vi "Read Is Server.vi"(8 "error in (no error)":errorcluster, 11 "WebSocket Server in":refnum<class "WebSocket Server.lvclass">) -> (0 "error out":errorcluster, 2 "Is Server?":bool, 3 "WebSocket Server out":refnum<class "WebSocket Server.lvclass">)   [LabVIEW 2013, in "WebSockets.lvlib" / "WebSocket Server.lvclass"]
uses:
  WebSocket Server.lvclass
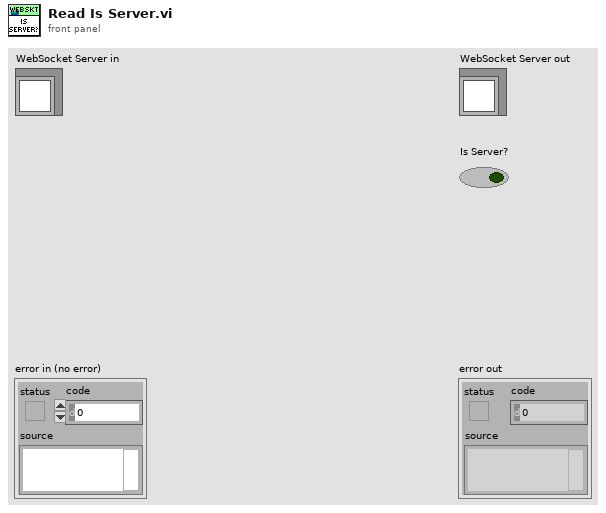
[diagram p1: front panel]
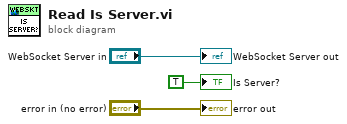
[diagram p0: block diagram]
diagram:
  "error out" <- "error in (no error)"
  "WebSocket Server out" <- "WebSocket Server in"
  "Is Server?" <- TRUE ("Is Server?")
